vi "getCscIndex.vi"(8 "error in (no error)":errorcluster, 11 "SalProcess in":refnum<class "SalProcess.lvclass">) -> (0 "error out":errorcluster, 2 "cscIdx":i32, 3 "SalProcess out":refnum<class "SalProcess.lvclass">)   [LabVIEW 2018, in "SalProcess.lvclass"]
doc: "Get the index of controlable SAL component (CSC)."
uses:
  SalProcess.lvclass
  <vilib>/Utility/config.llb/Read Key (I32).vi
  <vilib>/Utility/config.llb/NI_LVConfig.lvlib
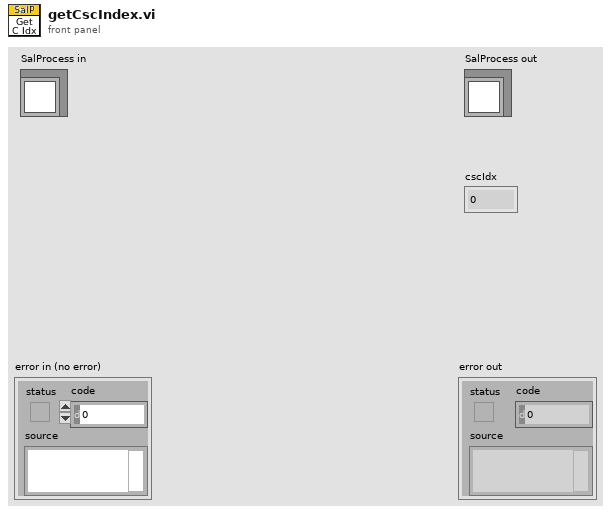
[diagram p1: front panel]
types:
  T1 = typedef "NI_LVConfig.lvlib/Config Data RefNum.ctl" = refnum<k1>
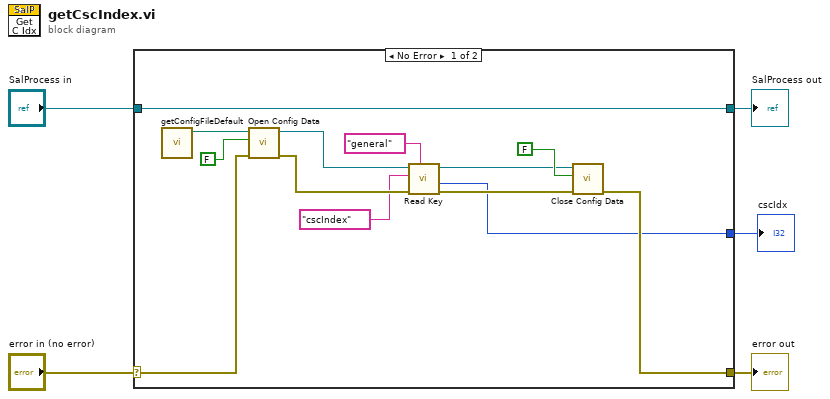
[diagram p0: block diagram]
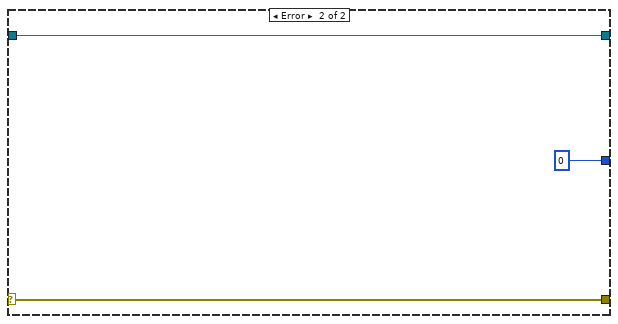
[diagram p2: hidden frame]
diagram:
  n1 = case shown="No Error" "error in (no error)" {
    selector: "error in (no error)" -> [w15 w21]
    tunnel: [w7 w21] -> w4
    tunnel: [w18 w20] -> w2
    tunnel: "SalProcess in" -> [w18 w20]
    tunnel: [w6 0 ("value")] -> w1
    frame No Error {
      n2 = call "getConfigFileDefault.vi"() -> ("configFileDefault"=w17:path)  [unwired: 11 in]
      n3 = call <vilib>:"Open Config Data.vi"("error in (no error)"=w15, "create file if necessary (T)"=FALSE, "configuration file path"=w17) -> ("error out"=w14:errorcluster, "refnum"=w10:T1)  [unwired: 6 in, 1 out]
      n4 = call-poly <vilib>:"Read Key.vi"("section"="general", "error in (no error)"=w14, "key"="cscIndex", "refnum"=w10) -> ("error out"=w8:errorcluster, "value"=w6:i32, "refnum out"=w9:T1)  [unwired: 4 in, 1 out]
      n5 = call <vilib>:"Close Config Data.vi"("error in (no error)"=w8, "write file if changed (T)"=FALSE, "refnum"=w9) -> ("error out"=w7:errorcluster)  [unwired: 7 in, 1 out]
    }
    frame Error {
    }
  }
  "error out" <- w4
  "SalProcess out" <- w2
  "cscIdx" <- w1
